vi "Database_OpenConnection.vi"(2 "error in":errorcluster, 3 "Database":string) -> (0 "error out":errorcluster, 1 "connection reference":T1)   [LabVIEW 2015]
uses:
  <vilib>/addons/database/Connection.llb/Conn ObjectReference.ctl
  <vilib>/addons/database/Connection.llb/DB Tools Open Connec (String).vi
  <vilib>/addons/database/NI_Database_API.lvlib
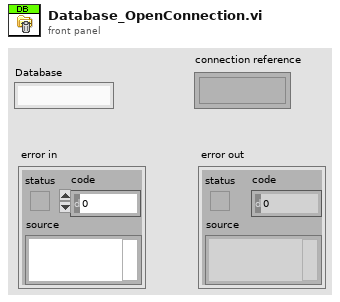
[diagram p1: front panel]
types:
  T1 = typedef "NI_Database_API.lvlib/Conn ObjectReference.ctl" = refnum<k1>
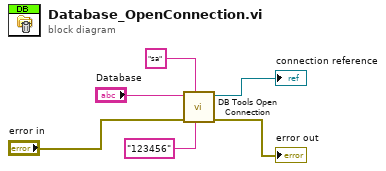
[diagram p0: block diagram]
diagram:
  n1 = call-poly <vilib>:"DB Tools Open Connection.vi"("password"="123456", "userID"="sa", "error in (no error)"="error in", "connection information"="Database") -> ("error out"=→"error out":errorcluster, "connection reference"=→"connection reference":T1)  [unwired: 4 in]
